vi "Initialize Controls.vi"(8 "error in":errorcluster, 11 "VI refnum in":refnum<vi>) -> (0 "error out":errorcluster, 3 "VI refnum out":refnum<vi>)   [LabVIEW 2018]
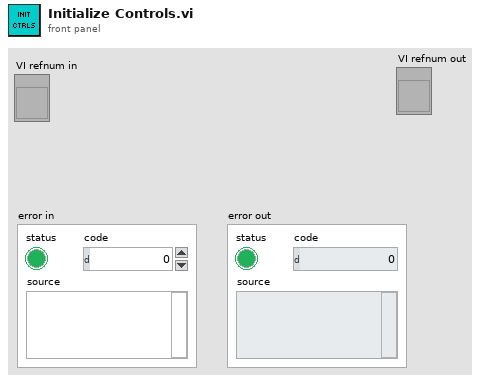
[diagram p1: front panel]
types:
  T1 = enum8{"Enabled", "Disabled", "Disabled and Grayed Out"}
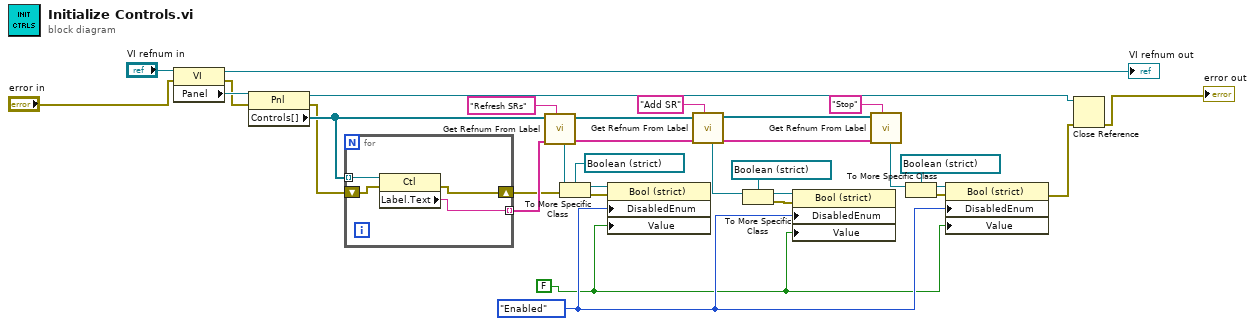
[diagram p0: block diagram]
diagram:
  w8 = FALSE ("Refresh SRs")
  w12 = T1."Enabled" ("Disabled")
  n1 = property class="VI"(reference="VI refnum in", error in="error in") -> (reference out=→"VI refnum out":refnum<vi>, error out=w31:errorcluster, "Panel"=w32:refnum<vi>)
  n2 = property class="Pnl"(reference=w32, error in=w31) -> (reference out=w4:refnum<vi>, error out=w29:errorcluster, "Controls[]"=w30:refnum<vi>[])
  n3 = for {
    tunnel: w30 -> [w37] mode=indexing
    shift-right: [w35] -> w24
    shift-left: w29 -> [w36]
    tunnel: [w34] -> w28 mode=indexing
    n4 = property class="Ctl"(reference=w37, error in=w36) -> (error out=w35:errorcluster, "Label.Text"=w34:string)  [unwired: 1 out]
  }
  n5 = call "Get Refnum From Label.vi"("label"="Refresh SRs", "label array in"=w28, "controls[] in"=w30) -> ("label array out"=w19:string[], "controls[] out"=w20:refnum<vi>[], "refnum out"=w27:refnum<vi>)  [unwired: 6 in]
  n6 = To More Specific Class(target class=refnum<vi> refnum ("reference"), reference=w27, error in=w24) -> (specific class reference=w26:refnum<vi>, error out=w25:errorcluster)
  n7 = property on="Property Node" class="Bool (strict)"(reference=w26, error in=w25, "DisabledEnum"=w12, "Value"=w8) -> ()  [unwired: 2 out]
  n8 = call "Get Refnum From Label.vi"("label"="Add SR", "label array in"=w19, "controls[] in"=w20) -> ("label array out"=w10:string[], "controls[] out"=w9:refnum<vi>[], "refnum out"=w21:refnum<vi>)  [unwired: 6 in]
  n9 = To More Specific Class(target class=refnum<vi> refnum ("reference"), reference=w21) -> (specific class reference=w22:refnum<vi>, error out=w23:errorcluster)  [unwired: 1 in]
  n10 = property on="Property Node" class="Bool (strict)"(reference=w22, error in=w23, "DisabledEnum"=w12, "Value"=w8) -> ()  [unwired: 2 out]
  n11 = call "Get Refnum From Label.vi"("label"="Stop", "label array in"=w10, "controls[] in"=w9) -> ("refnum out"=w18:refnum<vi>)  [unwired: 6 in, 2 out]
  n12 = To More Specific Class(target class=refnum<vi> refnum ("reference"), reference=w18) -> (specific class reference=w17:refnum<vi>, error out=w16:errorcluster)  [unwired: 1 in]
  n13 = property on="Property Node" class="Bool (strict)"(reference=w17, error in=w16, "DisabledEnum"=w12, "Value"=w8) -> (error out=w3:errorcluster)  [unwired: 1 out]
  n14 = Close Reference(reference=w4, error in (no error)=w3) -> (error out=→"error out":errorcluster)
